vi "Configure Marker State.vi"(7 "Maker On (F)":bool, 8 "error in (no error)":errorcluster, 10 "Marker Number (1)":u32=1 min=1, 11 "MXA in":refnum<class "MXA.lvclass">) -> (0 "error out":errorcluster, 3 "MXA out":refnum<class "MXA.lvclass">)   [LabVIEW 2020, in "MXA.lvclass"]
uses:
  MXA.lvclass
  C:/Sandbox/Git_Sandbox/WiSpry Test Framework source code (LV20)/WiSpry Test Framework/Instruments/Instrument.lvclass
  Instrument.lvclass/Instrument.ctl
  <instrlib>/Agilent MXA Series/Public/Configure/Marker/Configure Marker Type (Swept SA).vi
  Instrument.lvclass
  <instrlib>/Agilent MXA Series/Agilent MXA Series.lvlib
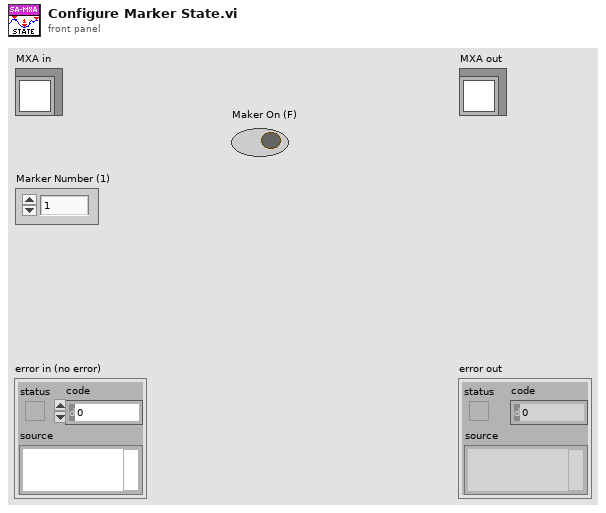
[diagram p1: front panel]
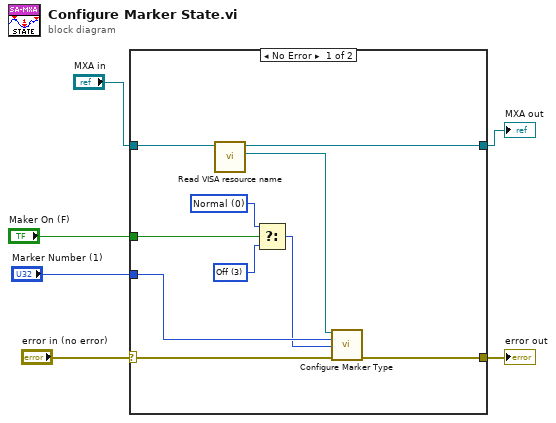
[diagram p0: block diagram]
diagram:
  n1 = case shown="No Error" "error in (no error)" {
    selector: "error in (no error)" -> [w12 w18]
    tunnel: "MXA in" -> [w16 w17]
    tunnel: [w11 w18] -> w5
    tunnel: [w15 w17] -> w4
    tunnel: "Marker Number (1)" -> [w13 _]
    tunnel: "Maker On (F)" -> [w9 _]
    frame No Error {
      w8 = 3 items=["Normal", "Delta", "Fixed", "Off"] ("Marker Type (0: Normal)")
      w10 = 0 items=["Normal", "Delta", "Fixed", "Off"] ("Marker Type (0: Normal)")
      n2 = call "Read VISA resource name.vi"("Instrument in"=w16) -> ("VISA resource name"=w14:refnum<visa-resource-name>, "Instrument out"=w15:refnum<class "MXA.lvclass">)  [unwired: 9 in]
      n3 = Select(t=w10, s=w9, f=w8) -> (s? t:f=w7:i32)
      n4 = call-poly <instrlib>:"Configure Marker Type.vi"("VISA resource name"=w14, "Active Marker (1: Marker1)"=w13, "Marker Type (0: Normal)"=w7, "error in (no error)"=w12) -> ("error out"=w11:errorcluster)  [unwired: 10 in, 1 out]
    }
    frame Error {
    }
  }
  "error out" <- w5
  "MXA out" <- w4
